vi "Encoder Movement.vi"(6 "STOP?":bool, 7 "Enc":dbl, 8 "error in":errorcluster, 9 "Speed":dbl, 10 "Move":T2(ring), 11 "FPGA VI Reference Out 2":refnum<k20>) -> (0 "error out":errorcluster, 2 "STOP NOW":bool, 3 "FPGA VI Reference Out":refnum<k20>)   [LabVIEW 2019]
uses:
  <vilib>/robotics/Steering/Mecanum Wheel/Roller Orientation.ctl
  <vilib>/robotics/Steering/Wheel/Wheel Parameters.ctl
  <vilib>/robotics/Steering/Wheel/Rotation Direction.ctl
  <vilib>/robotics/Steering/Mecanum Steering Frame/NI_Robotics_Mecanum Steering Frame.lvclass
  C:/Program Files (x86)/National Instruments/LabVIEW 2019/vi.lib/robotics/Steering/Steering Frame/NI_Robotics_Steering Frame.lvclass
  <vilib>/robotics/Steering/Mecanum Wheel/Create Mecanum Wheel.vi
  <vilib>/robotics/Steering/Mecanum Steering Frame/Create Mecanum Steering Frame.vi
  <vilib>/Utility/error.llb/Error Cluster From Error Code.vi
  <vilib>/rvi/errors/niLvFpgaAdjustHostInterfaceError.vi
  <vilib>/robotics/Steering/Steering Frame/Apply Steering Frame Velocity to Motors.vi
  <vilib>/robotics/Steering/Create Steering Frame/NI_Robotics_Create Steering Frame.xnode
  <vilib>/robotics/Steering/Class Type Definitions/Mecanum Steering Frame.ctl
  <vilib>/rvi/interface/nirviReadWriteControl/nirviReadWriteControl.xnode
  <vilib>/robotics/Steering/Class Type Definitions/NI_Robotics_Steering Class Types.lvlib
  <vilib>/robotics/Steering/Steering Frame/NI_Robotics_Steering Frame.lvclass
  NiFpgaLv.dll
  <vilib>/rvi/interface/Simulation/niFpgaSimulationCallBeginRW.vi
  <vilib>/robotics/Steering/Mecanum Wheel/NI_Robotics_Mecanum Wheel.lvclass
  <vilib>/robotics/Steering/Wheel/NI_Robotics_Wheel.lvclass
  <vilib>/rvi/interface/nirviOpenFPGA/nirviOpenFPGA.xnode
  Collin's Project/FPGA Bitfiles/MRmecanum_FPGATarget_FPGAMainModified_TerasRobot_LKSN2021.lvbitx
  <vilib>/FPGAPlugInAG/myRIO-1900/niLvFpga_Open_myRIO-1900.vi
  <vilib>/rvi/interface/common/dynamic/niFpgaDynamicAddResources.vi
  <vilib>/rvi/interface/nirviCloseFPGA/nirviCloseFPGA.xnode
  <vilib>/FPGAPlugInAG/Dynamic/niLvFpga_Close_Dynamic.vi
  C:/Program Files (x86)/National Instruments/LabVIEW 2019/vi.lib/robotics/Steering/Special Steering Frame/NI_Robotics_Special Steering Frame.lvclass
panel:
  out "ENC M4":i32
  out "ENC M3":i32
  out "ENC M2":i32
  out "ENC M1":i32
  in  "error in 2":errorcluster
  out "error out 2":errorcluster
  in  "Enum":T1(ring)=enum."none"
  out "ENC M5 2":i32
  in  "Negate?":bool
  out "ENC M5 3":i32
  out "ENC M5":i32
  out "Encoder":i32
  in  "FPGA VI Reference Out 4":refnum<k20>
  out "FPGA VI Reference Out 3":refnum<k20>
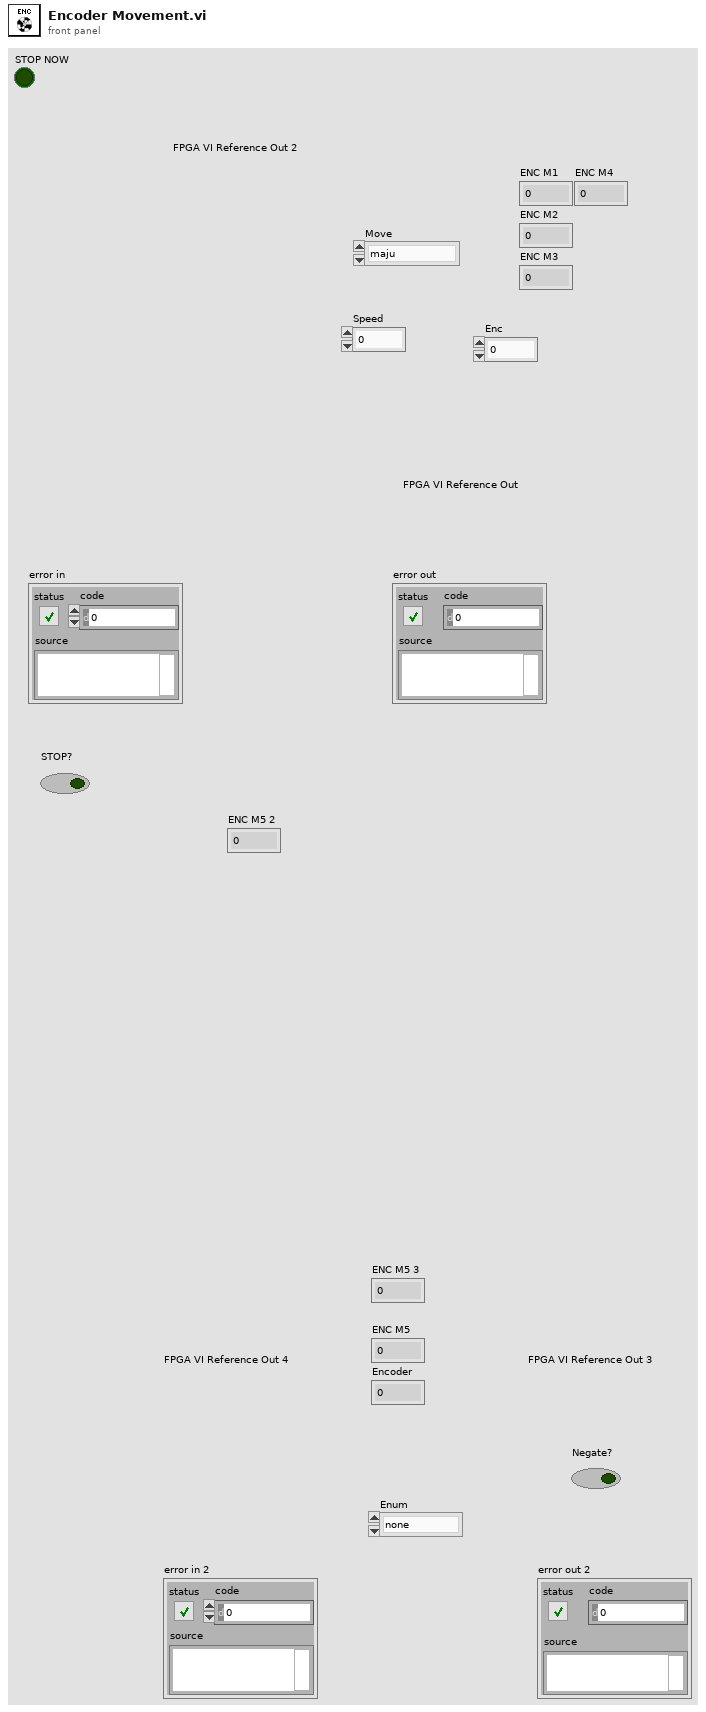
[diagram p1: front panel]
types:
  T1 = enum16{"top to mid", "mid to down", "top to down", "none"}
  T2 = enum16{"maju", "mundur", "kanan", "kiri", "atas kanan", "atas kiri", "bawah kanan", "bawah kiri", "putar kanan", "putar kiri"}
  T3 = typedef "NI_Robotics_Steering Class Types.lvlib/Mecanum Steering Frame.ctl" = refnum<class "NI_Robotics_Mecanum Steering Frame.lvclass">
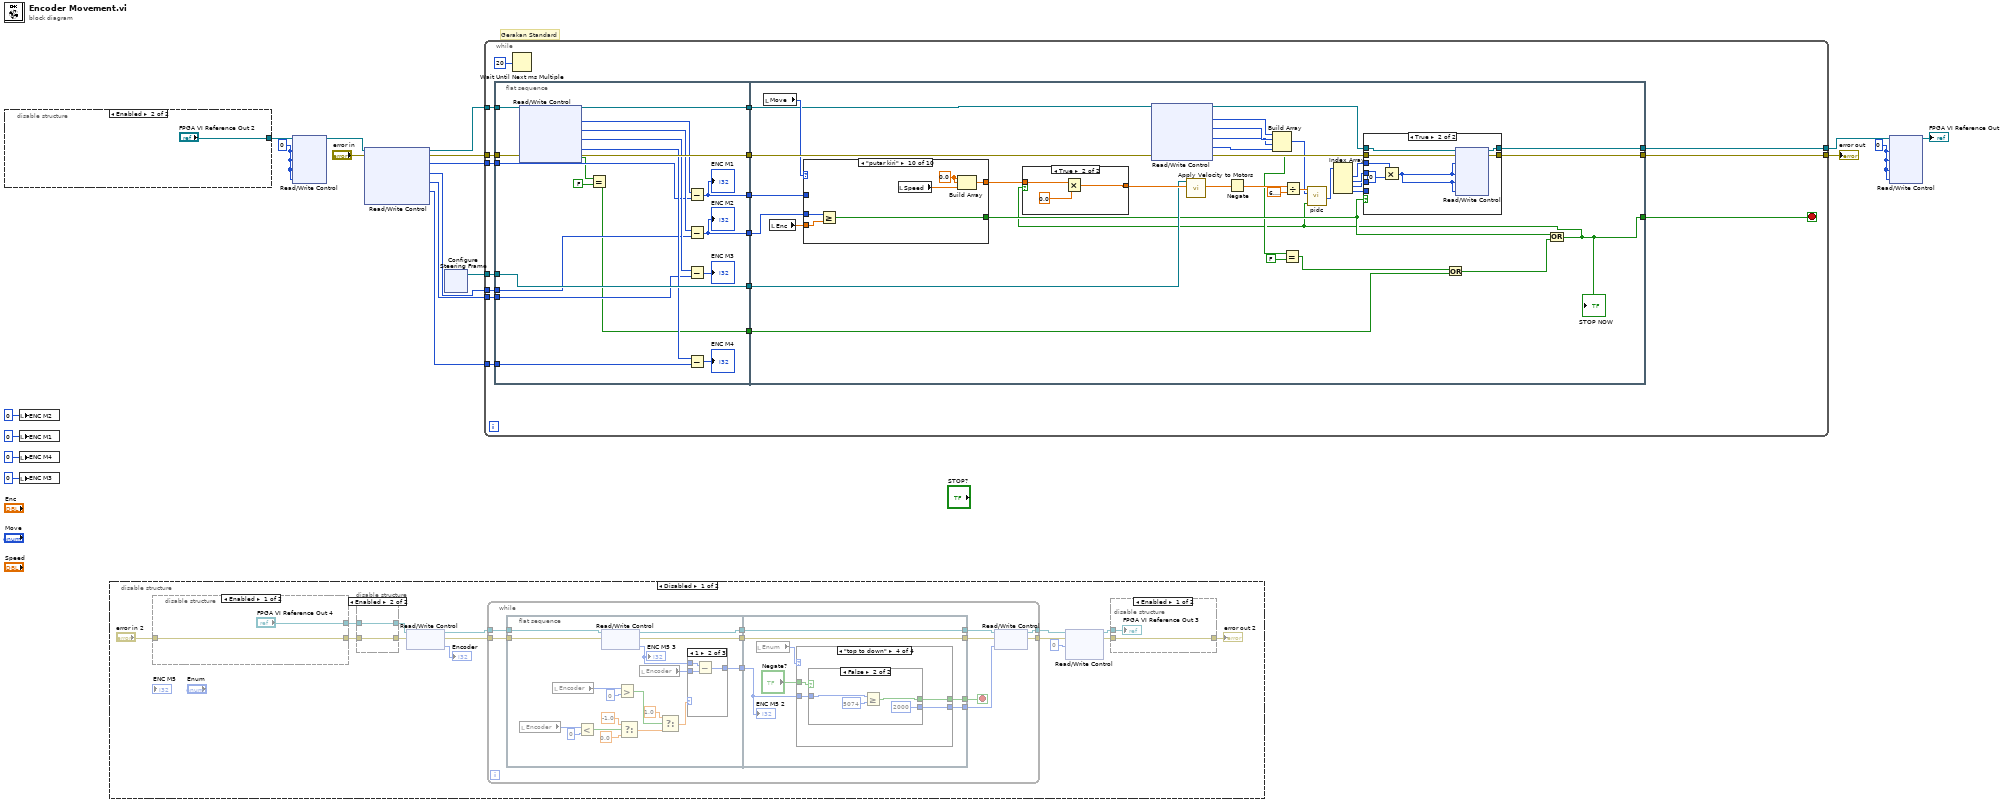
[diagram p0: block diagram]
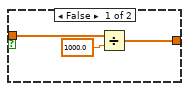
[diagram p2: hidden frame]
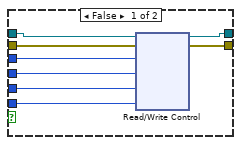
[diagram p3: hidden frame]
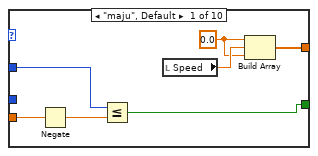
[diagram p4: hidden frame]
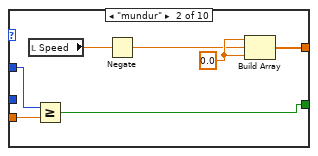
[diagram p5: hidden frame]
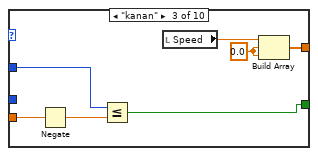
[diagram p6: hidden frame]
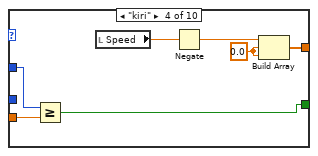
[diagram p7: hidden frame]
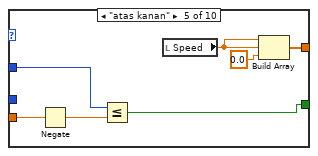
[diagram p8: hidden frame]
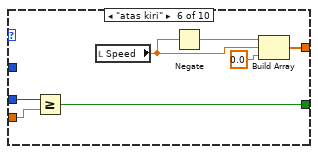
[diagram p9: hidden frame]
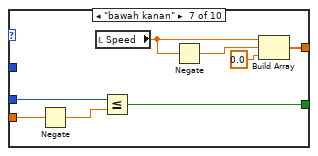
[diagram p10: hidden frame]
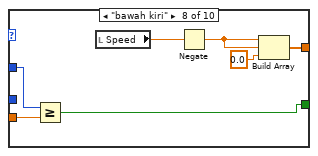
[diagram p11: hidden frame]
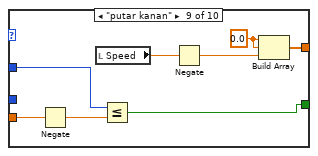
[diagram p12: hidden frame]
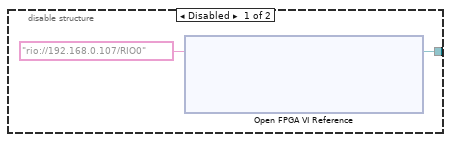
[diagram p13: hidden frame]
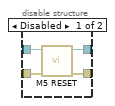
[diagram p14: hidden frame]
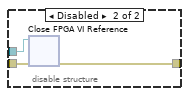
[diagram p15: hidden frame]
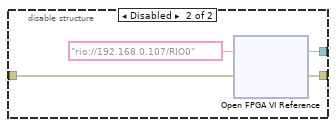
[diagram p16: hidden frame]
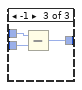
[diagram p18: hidden frame]
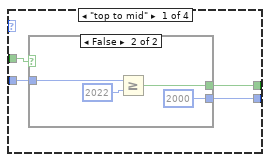
[diagram p19: hidden frame]
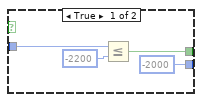
[diagram p20: hidden frame]
diagram:
  w2 = i16 0 ("M1")
  w8 = i16 0 ("M1")
  # "Gerakan Standard"
  n1 = disable-structure shown="Enabled" {
    disable-tunnel: [w20 "FPGA VI Reference Out 2"] -> w7
    frame Disabled {
      n2 = xnode "Open FPGA VI Reference"("resource name"=tag "rio://192.168.0.107/RIO0") -> ("FPGA VI Reference Out"=w20:refnum<k20>)  [unwired: 1 in, 1 out]
    }
    frame Enabled {
    }
  }
  n3 = local write "ENC M2"(0 ("ENC M2 2")) -> ()
  n4 = local write "ENC M1"(0 ("ENC M1 2")) -> ()
  n5 = local write "ENC M4"(0 ("ENC M4 2")) -> ()
  n6 = local write "ENC M3"(0 ("ENC M3 2")) -> ()
  n7 = disable-structure shown="Disabled" {
    frame Disabled {
      n8 = disable-structure shown="Enabled" {
        disable-tunnel: ["FPGA VI Reference Out 4" w52] -> w33
        disable-tunnel: [w48 w51] -> w36
        disable-tunnel: "error in 2" -> [w48 w50]
        frame Enabled {
        }
        frame Disabled {
          n9 = xnode "Open FPGA VI Reference"("error in"=w50, "resource name"=tag "rio://192.168.0.107/RIO0") -> ("FPGA VI Reference Out"=w52:refnum<k20>, "error out"=w51:errorcluster)
        }
      }
      n10 = disable-structure shown="Enabled" {
        disable-tunnel: w33 -> [w40 w42]
        disable-tunnel: [w39 w42] -> w34
        disable-tunnel: [w38 w41] -> w35
        disable-tunnel: w36 -> [w37 w41]
        frame Disabled {
          n11 = call "M5 RESET.vi"("FPGA VI Reference Out"=w40, "error in"=w37) -> ("FPGA VI Reference Out"=w39:refnum<k20>, "error out"=w38:errorcluster)  [unwired: 7 in]
        }
        frame Enabled {
        }
      }
      n12 = xnode "Read/Write Control"("FPGA VI Reference In"=w34, "error in"=w35) -> ("FPGA VI Reference Out"=w26:refnum<k20>, "error out"=w27:errorcluster, "ENC M5"=→"Encoder":i32)
      n13 = while {
        tunnel: [w62] -> w23
        tunnel: [w61] -> w24
        tunnel: w26 -> [w60]
        tunnel: w27 -> [w59]
        stop <- w54 stop-if-true
        n14 = flat-sequence {
          tunnel: w60 -> [w80]
          tunnel: w59 -> [w79]
          tunnel: [w82] -> w58
          tunnel: [w81] -> w57
          tunnel: [w65] -> w56
          tunnel: [w95] -> w63
          tunnel: [w96] -> w64
          tunnel: w58 -> [w96]
          tunnel: w57 -> [w95]
          tunnel: w56 -> [w93]
          tunnel: [w92] -> w55
          tunnel: [w91] -> w54
          frame #0 {
            n15 = local read "Encoder"() -> (w74:i32)
            n16 = local read "Encoder"() -> (w78:i32)
            n17 = Less?(x=w74, y=0) -> (x < y?=w72:bool)
            n18 = xnode "Read/Write Control"("FPGA VI Reference In"=w80, "error in"=w79) -> ("FPGA VI Reference Out"=w82:refnum<k20>, "error out"=w81:errorcluster, "ENC M5"=w66:i32)
            "ENC M5 3" <- w66
            n19 = Greater?(x=w78, y=0) -> (0:w76:bool)
            n20 = Select(t=-1.0, s=w72, f=0.0) -> (s? t:f=w71:dbl)
            n21 = local read "Encoder"() -> (w67:i32)
            n22 = Select(t=1.0, s=w76, f=w71) -> (s? t:f=w68:dbl)
            n23 = case shown="1" w68 {
              tunnel: w67 -> [_ w86 w89]
              tunnel: w66 -> [w83 w85 w88]
              tunnel: [w83 w84 w87] -> w65
              frame 0, Default {
              }
              frame 1 {
                n24 = Subtract(x=w85, y=w86) -> (x-y=w84:i32)
              }
              frame -1 {
                n25 = Subtract(x=w88, y=w89) -> (x-y=w87:i32)
              }
            }
          }
          frame #1 {
            n26 = local read "Enum"() -> (w94:T1)
            n27 = case shown="\"top to down\"" w94 {
              tunnel: [w100 w112 i16 0 ("M5") w128] -> w92
              tunnel: [w98 w110 w123 w126] -> w91
              tunnel: w93 -> [w99 w111 w122 w127]
              tunnel: "Negate?" -> [w97 w109 _ w125]
              frame "top to mid" {
                n28 = case shown="False" w97 {
                  tunnel: [i16 -2000 ("M5") i16 2000 ("M5")] -> w100
                  tunnel: w99 -> [w103 w107]
                  tunnel: [w102 w106] -> w98
                  frame True {
                    n29 = Less Or Equal?(x=w103, y=-2200) -> (x <= y?=w102:bool)
                  }
                  frame False {
                    n30 = Greater Or Equal?(x=w107, y=2022) -> (x >= y?=w106:bool)
                  }
                }
              }
              frame "mid to down" {
                n31 = case shown="False" w109 {
                  tunnel: [i16 -2000 ("M5") i16 2000 ("M5")] -> w112
                  tunnel: w111 -> [w115 w119]
                  tunnel: [w114 w118] -> w110
                  frame True {
                    n32 = Less Or Equal?(x=w115, y=-2630) -> (x <= y?=w114:bool)
                  }
                  frame False {
                    n33 = Greater Or Equal?(x=w119, y=2630) -> (x >= y?=w118:bool)
                  }
                }
              }
              frame "none", Default {
                n34 = Equal?(x=w122, y=0) -> (x = y?=w123:bool)
              }
              frame "top to down" {
                n35 = case shown="False" w125 {
                  tunnel: [i16 -2000 ("M5") i16 2000 ("M5")] -> w128
                  tunnel: w127 -> [w131 w135]
                  tunnel: [w130 w134] -> w126
                  frame True {
                    n36 = Less Or Equal?(x=w131, y=-5074) -> (x <= y?=w130:bool)
                  }
                  frame False {
                    n37 = Greater Or Equal?(x=w135, y=5074) -> (x >= y?=w134:bool)
                  }
                }
              }
            }
            "ENC M5 2" <- w93
          }
        }
        n38 = xnode "Read/Write Control"("FPGA VI Reference In"=w64, "error in"=w63, "M5"=w55) -> ("FPGA VI Reference Out"=w62:refnum<k20>, "error out"=w61:errorcluster)
      }
      n39 = xnode "Read/Write Control"("FPGA VI Reference In"=w23, "error in"=w24, "M5"=i16 0) -> ("FPGA VI Reference Out"=w30:refnum<k20>, "error out"=w31:errorcluster)  [unwired: 1 out]
      n40 = disable-structure shown="Enabled" {
        disable-tunnel: w30 -> [w44 w47]
        disable-tunnel: w31 -> [w43 w46]
        disable-tunnel: [w43 w45] -> w32
        frame Enabled {
          "FPGA VI Reference Out 3" <- w44
        }
        frame Disabled {
          n41 = xnode "Close FPGA VI Reference"("FPGA VI Reference In"=w47, "error in"=w46) -> ("error out"=w45:errorcluster)
        }
      }
      "error out 2" <- w32
    }
    frame Enabled {
    }
  }
  n42 = xnode "Read/Write Control"("FPGA VI Reference In"=w7, "M1"=w8, "M2"=w8, "M3"=w8, "M4"=w8) -> ("FPGA VI Reference Out"=w6:refnum<k20>)  [unwired: 1 in, 1 out]
  n43 = xnode "Read/Write Control"("FPGA VI Reference In"=w6, "error in"="error in") -> ("FPGA VI Reference Out"=w19:refnum<k20>, "error out"=w18:errorcluster, "ENC M1"=w17:i32, "ENC M2"=w16:i32, "ENC M3"=w15:i32, "ENC M4"=w14:i32)  [unwired: 1 in]
  n44 = xnode ("Configure Steering Frame")() -> ("mecanum steering frame out"=w1:T3)  [unwired: 1 in, 1 out]
  n45 = while {
    tunnel: w19 -> [w142]
    tunnel: [w153] -> w4
    tunnel: w18 -> [w151]
    tunnel: [w152] -> w5
    tunnel: w1 -> [w150]
    tunnel: w17 -> [w143]
    tunnel: w16 -> [w144]
    tunnel: w15 -> [w145]
    tunnel: w14 -> [w146]
    stop <- w140 stop-if-true
    n46 = flat-sequence {
      tunnel: w150 -> [w171]
      tunnel: w151 -> [w172]
      tunnel: [w172] -> w149
      tunnel: [w164] -> w148
      tunnel: [w171] -> w147
      tunnel: w146 -> [w163]
      tunnel: w145 -> [w162]
      tunnel: w144 -> [w161]
      tunnel: w143 -> [w160]
      tunnel: w142 -> [w159]
      tunnel: [w158] -> w141
      tunnel: [w157] -> w139
      tunnel: [w154] -> w137
      tunnel: [w179] -> w153
      tunnel: [w205] -> w152
      tunnel: w149 -> [w204]
      tunnel: w148 -> [w194]
      tunnel: w147 -> [w193]
      tunnel: w141 -> [w184]
      tunnel: [w173] -> w140
      tunnel: w139 -> [w181]
      tunnel: w137 -> [w175]
      frame #0 {
        n47 = xnode "Read/Write Control"("FPGA VI Reference In"=w159) -> ("FPGA VI Reference Out"=w164:refnum<k20>, "ENC M1"=w165:i32, "ENC M2"=w166:i32, "ENC M3"=w167:i32, "ENC M4"=w168:i32, "START BUTTON"=w156:bool)  [unwired: 1 in, 1 out]
        n48 = Equal?(x=w156, y=FALSE) -> (x = y?=w154:bool)
        n49 = Subtract(x=w165, y=w160) -> (x-y=w158:i32)
        "ENC M1" <- w158
        n50 = Subtract(x=w166, y=w161) -> (x-y=w157:i32)
        "ENC M2" <- w157
        n51 = Subtract(x=w167, y=w162) -> (x-y=→"ENC M3":i32)
        n52 = Subtract(x=w168, y=w163) -> (x-y=→"ENC M4":i32)
      }
      frame #1 {
        n53 = local read "Move"() -> (w203:T2)
        n54 = local read "Enc"() -> (w183:dbl)
        n55 = case shown="\"putar kiri\"" w203 {
          tunnel: [w231 w238 w246 w253 w260 w268 w276 w283 w289 w296] -> w192
          tunnel: w184 -> [w230 w235 w244 w250 w258 _ _ w278 w287 _]
          tunnel: w183 -> [w229 w236 w243 w249 w257 w263 w272 w279 w288 w292]
          tunnel: [w228 w234 w242 w248 w256 w264 w271 w277 w285 w295] -> w180
          tunnel: w181 -> [_ _ _ _ _ w262 w269 _ _ w293]
          frame "maju", Default {
            w232 = 0.0 ("element")
            n56 = Negate(x=w229) -> (-x=w227:dbl)
            n57 = Less Or Equal?(x=w230, y=w227) -> (x <= y?=w228:bool)
            n58 = local read "Speed"() -> (w233:dbl)
            n59 = Build Array(w232, w233, w232) -> (w231:dbl[])
          }
          frame "mundur" {
            w239 = 0.0 ("element")
            n60 = local read "Speed"() -> (w240:dbl)
            n61 = Greater Or Equal?(x=w235, y=w236) -> (x >= y?=w234:bool)
            n62 = Negate(x=w240) -> (-x=w237:dbl)
            n63 = Build Array(w239, w237, w239) -> (w238:dbl[])
          }
          frame "kanan" {
            w245 = 0.0 ("element")
            n64 = Negate(x=w243) -> (-x=w241:dbl)
            n65 = Less Or Equal?(x=w244, y=w241) -> (x <= y?=w242:bool)
            n66 = local read "Speed"() -> (w247:dbl)
            n67 = Build Array(w247, w245, w245) -> (w246:dbl[])
          }
          frame "kiri" {
            w251 = 0.0 ("element")
            n68 = Greater Or Equal?(x=w250, y=w249) -> (x >= y?=w248:bool)
            n69 = local read "Speed"() -> (w254:dbl)
            n70 = Negate(x=w254) -> (-x=w252:dbl)
            n71 = Build Array(w252, w251, w251) -> (w253:dbl[])
          }
          frame "atas kanan" {
            n72 = Negate(x=w257) -> (-x=w255:dbl)
            n73 = Less Or Equal?(x=w258, y=w255) -> (x <= y?=w256:bool)
            n74 = local read "Speed"() -> (w261:dbl)
            n75 = Build Array(w261, w261, 0.0 ("element")) -> (w260:dbl[])
          }
          frame "atas kiri" {
            n76 = Greater Or Equal?(x=w262, y=w263) -> (x >= y?=w264:bool)
            n77 = local read "Speed"() -> (w265:dbl)
            n78 = Negate(x=w265) -> (-x=w266:dbl)
            n79 = Build Array(w266, w265, 0.0 ("element")) -> (w268:dbl[])
          }
          frame "bawah kanan" {
            n80 = Negate(x=w272) -> (-x=w270:dbl)
            n81 = local read "Speed"() -> (w273:dbl)
            n82 = Less Or Equal?(x=w269, y=w270) -> (x <= y?=w271:bool)
            n83 = Negate(x=w273) -> (-x=w274:dbl)
            n84 = Build Array(w273, w274, 0.0 ("element")) -> (w276:dbl[])
          }
          frame "bawah kiri" {
            n85 = Greater Or Equal?(x=w278, y=w279) -> (x >= y?=w277:bool)
            n86 = local read "Speed"() -> (w281:dbl)
            n87 = Negate(x=w281) -> (-x=w280:dbl)
            n88 = Build Array(w280, w280, 0.0 ("element")) -> (w283:dbl[])
          }
          frame "putar kanan" {
            w291 = 0.0 ("element")
            n89 = Negate(x=w288) -> (-x=w286:dbl)
            n90 = local read "Speed"() -> (w290:dbl)
            n91 = Less Or Equal?(x=w287, y=w286) -> (x <= y?=w285:bool)
            n92 = Negate(x=w290) -> (-x=w284:dbl)
            n93 = Build Array(w291, w291, w284) -> (w289:dbl[])
          }
          frame "putar kiri" {
            w297 = 0.0 ("element")
            n94 = Greater Or Equal?(x=w293, y=w292) -> (x >= y?=w295:bool)
            n95 = local read "Speed"() -> (w294:dbl)
            n96 = Build Array(w297, w297, w294) -> (w296:dbl[])
          }
        }
        n97 = xnode "Read/Write Control"("FPGA VI Reference In"=w194) -> ("FPGA VI Reference Out"=w182:refnum<k20>, "ENC M1"=w189:i32, "ENC M2"=w188:i32, "ENC M3"=w187:i32, "ENC M4"=w186:i32, "START BUTTON"=w178:bool)  [unwired: 1 in, 1 out]
        n98 = Build Array(w189, w188, w187, w186) -> (w185:i32[])
        n99 = Equal?(x=w178, y=FALSE) -> (x = y?=w176:bool)
        n100 = Or(x=w176, y=w175) -> (x .or. y?=w174:bool)
        n101 = Or(x=w180, y=w174) -> (x .or. y?=w173:bool)
        "STOP NOW" <- w173
        n102 = case shown="True" w173 {
          tunnel: [w207 w209] -> w195
          tunnel: w192 -> [w206 w211]
          frame False {
            n103 = Divide(x=w206, y=1000.0) -> (x/y=w207:dbl[])
          }
          frame True {
            n104 = Multiply(x=w211, y=0.0) -> (x*y=w209:dbl[])
          }
        }
        n105 = call-poly <vilib>:"Apply Velocity to Motors.vi"("steering frame velocity"=w195, "steering frame in"=w193) -> ("ccw motor velocity setpoints"=w191:dbl[])  [unwired: 5 in, 4 out]
        n106 = Negate(x=w191) -> (-x=w202:dbl[])
        n107 = Divide(x=w202, y=6.283185307179586) -> (x/y=w190:dbl[])
        n108 = call "pidc.vi"("Stop"=w173, "input encoder 2"=w185, "input rps"=w190) -> ("Output duty cycle"=w200:i16[])  [unwired: 8 in]
        n109 = Index Array(array=w200) -> (element #1=w199:i16, element #2=w198:i16, element #3=w197:i16, element #4=w196:i16)  [unwired: 4 in]
        n110 = case shown="True" w180 {
          tunnel: [w219 w226] -> w179
          tunnel: [w218 w225] -> w205
          tunnel: w204 -> [w217 w224]
          tunnel: w199 -> [w216 w222]
          tunnel: w198 -> [w215 _]
          tunnel: w197 -> [w214 _]
          tunnel: w196 -> [w213 _]
          tunnel: w182 -> [w212 w223]
          frame False {
            n111 = xnode "Read/Write Control"("FPGA VI Reference In"=w212, "error in"=w217, "M1"=w216, "M2"=w215, "M3"=w214, "M4"=w213) -> ("FPGA VI Reference Out"=w219:refnum<k20>, "error out"=w218:errorcluster)
          }
          frame True {
            n112 = Multiply(x=w222, y=i16 0) -> (x*y=w220:i16)
            n113 = xnode "Read/Write Control"("FPGA VI Reference In"=w223, "error in"=w224, "M1"=w220, "M2"=w220, "M3"=w220, "M4"=w220) -> ("FPGA VI Reference Out"=w226:refnum<k20>, "error out"=w225:errorcluster)
          }
        }
      }
    }
    n114 = Wait Until Next ms Multiple(millisecond multiple=u32 20) -> ()  [unwired: 1 out]
  }
  "error out" <- w5
  n115 = xnode "Read/Write Control"("FPGA VI Reference In"=w4, "M1"=w2, "M2"=w2, "M3"=w2, "M4"=w2) -> ("FPGA VI Reference Out"=→"FPGA VI Reference Out":refnum<k20>)  [unwired: 1 in, 1 out]
